vi "AcquireCameraImages.vi"() -> ()   [LabVIEW 2019]
uses:
  RecognitionResponse.ctl
  <vilib>/vision/Image Controls.llb/IMAQ Image.ctl
  <vilib>/vision/driver/IMAQdx.llb/IMAQdx Buffer Number Mode.ctl
  <vilib>/vision/driver/NI_Vision_Acquisition_Software.lvlib
panel:
  in  "Check face":bool
  out "error out":errorcluster
  out "Faces sent":i32
  out "value":T1={"probability"=0.0, "recognized_class"="127.0.0.1", "outcome"="false"}
  out "Image out":T2(plugin-control)
  out "Processing Frame Rate":dbl
  out "Acquired Frame Rate":dbl
  in  "Stop":bool
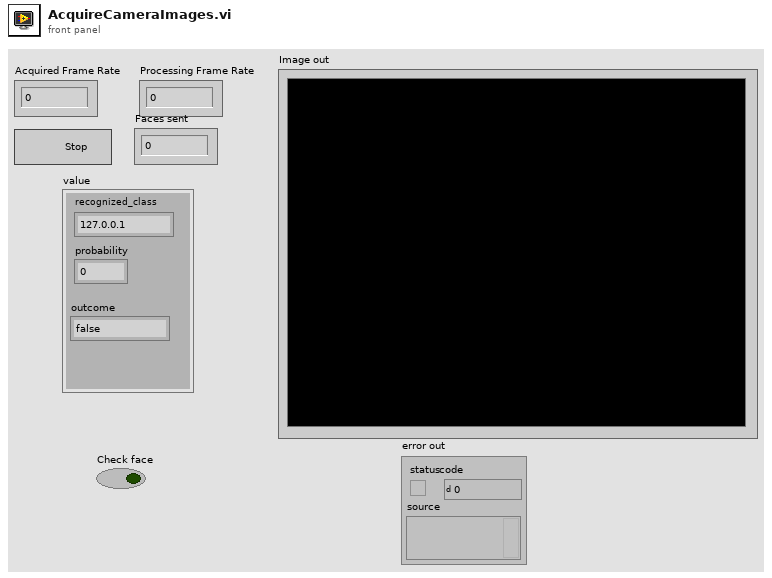
[diagram p1: front panel]
types:
  T1 = typedef "RecognitionResponse.ctl" = cluster{"probability":dbl, "recognized_class":string, "outcome":string}
  T2 = typedef "IMAQ Image.ctl" = refnum<image>
  T3 = typedef "IMAQ Object Tracking Session.ctl" = refnum<k20>
  T4 = typedef "IMAQdx.ctl" = refnum<k21>
  T5 = typedef "NI_Vision_Acquisition_Software.lvlib/IMAQdx Buffer Number Mode.ctl" = enum32{"Next", "Last", "Buffer Number", "Every", "Last New"}
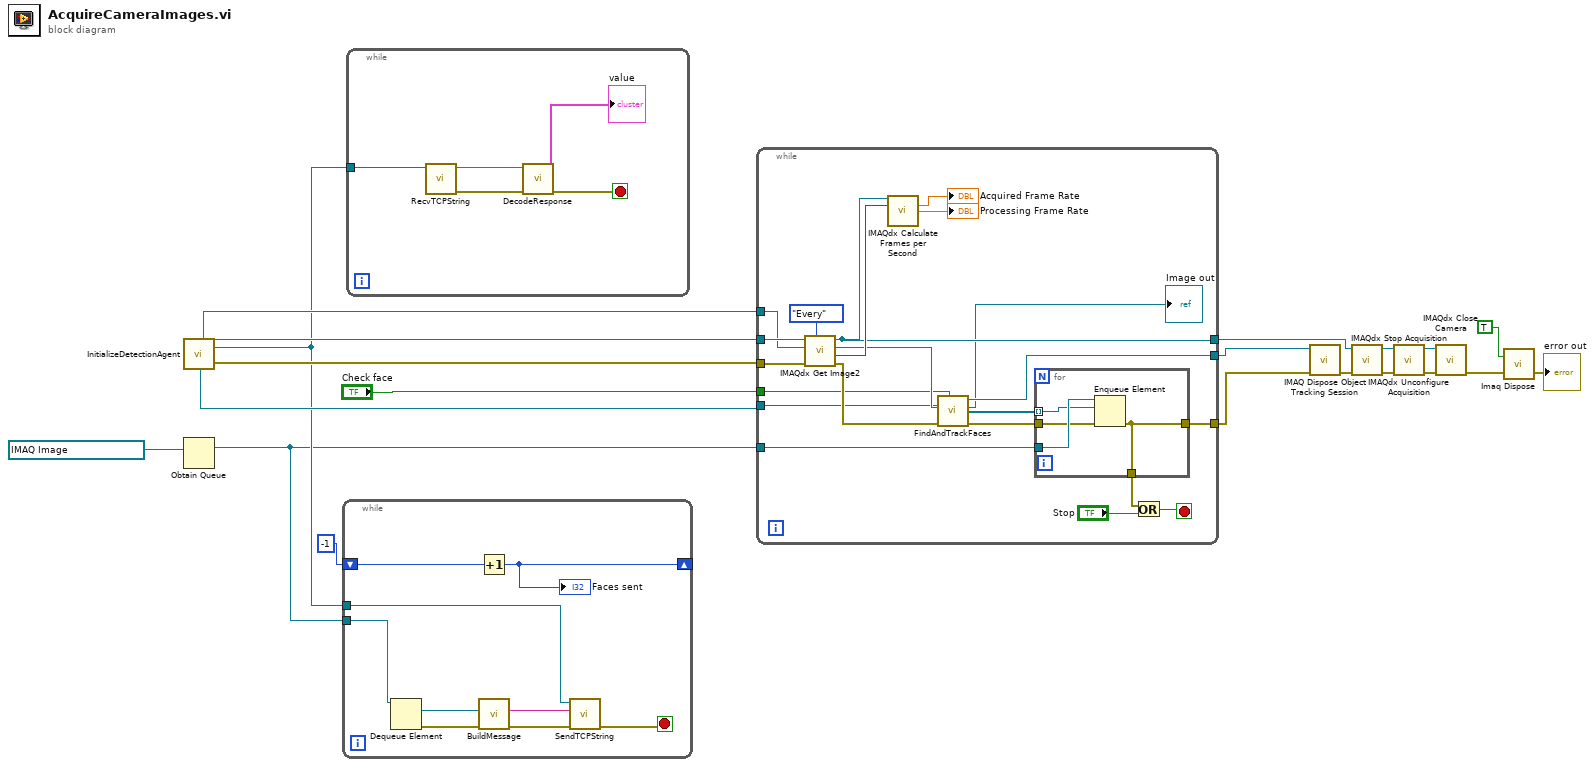
[diagram p0: block diagram]
diagram:
  n1 = call "InitializeDetectionAgent.vi"() -> ("error out"=w8:errorcluster, "Object Tracking Session Out"=w9:T3, "Session Out"=w10:T4, "connection ID"=w6:refnum<k5>, "Aquisition Image"=w11:T2)  [unwired: 6 in]
  n2 = Obtain Queue(element data type=T2 refnum ("Image type")) -> (queue out=w5:refnum<queue>)  [unwired: 4 in, 2 out]
  n3 = while {
    tunnel: w5 -> [w29]
    shift-right: [w21] -> _
    shift-left: -1 -> [w27]
    tunnel: w6 -> [w25]
    stop <- w22 stop-if-true
    n4 = Dequeue Element(queue=w29) -> (element=w28:T2, error out=w26:errorcluster)  [unwired: 2 in, 2 out]
    n5 = Increment(x=w27) -> (x+1=w21:i32)
    "Faces sent" <- w21
    n6 = call "BuildMessage.vi"("error in"=w26, "Image"=w28) -> ("error out"=w24:errorcluster, "JSON string"=w23:string)  [unwired: 7 in, 1 out]
    n7 = call "SendTCPString.vi"("error in (no error)"=w24, "String"=w23, "TCP Network Connection in"=w25) -> ("error out"=w22:errorcluster)  [unwired: 8 in]
  }
  n8 = while {
    tunnel: w6 -> [w32]
    stop <- w30 stop-if-true
    n9 = call "RecvTCPString.vi"("TCP Network Connection in"=w32) -> ("error out"=w31:errorcluster, "data out"=w34:string)  [unwired: 9 in]
    n10 = call "DecodeResponse.vi"("error in (no error)"=w31, "data in"=w34) -> ("error out"=w30:errorcluster, "RecognitionResponse"=→"value":T1)  [unwired: 8 in]
  }
  n11 = while {
    tunnel: [w50] -> w15
    tunnel: w8 -> [w55]
    tunnel: w10 -> [w54]
    tunnel: w11 -> [w52]
    tunnel: [w45] -> w13
    tunnel: w9 -> [w42]
    tunnel: w5 -> [w41]
    tunnel: [w39] -> w3
    tunnel: "Check face" -> [w35]
    stop <- w36 stop-if-true
    n12 = call <vilib>:"IMAQdx Get Image2.vi"("Buffer Number Mode (Next)"=IMAQdx_Buffer_Number_Mode."Every" ("Buffer Number Mode"), "error in"=w55, "Image In"=w52, "Session In"=w54) -> ("error out"=w46:errorcluster, "Buffer Number Out"=w51:u32, "Image Out"=w47:T2, "Session Out"=w50:T4)  [unwired: 4 in]
    n13 = call <vilib>:"IMAQdx Calculate Frames per Second.vi"("Session In"=w50, "Buffer Number"=w51) -> ("Acquired Frames per Second"=→"Acquired Frame Rate":dbl, "Processed Frames per Second"=→"Processing Frame Rate":dbl)  [unwired: 7 in, 5 out]
    n14 = call "FindAndTrackFaces.vi"("Check face"=w35, "error in (no error)"=w46, "Image in"=w47, "Object Tracking Session In"=w42) -> ("error out"=w43:errorcluster, "Face Images"=w44:T2[], "Image out"=→"Image out":T2, "Object Tracking Session Out"=w45:T3)  [unwired: 4 in]
    n15 = for {
      tunnel: w44 -> [w58] mode=indexing
      tunnel: w43 -> [w57]
      tunnel: w41 -> [w59]
      tunnel: [w56] -> w39
      tunnel: [w56] -> w37
      n16 = Enqueue Element(queue=w59, element=w58, error in (no error)=w57) -> (error out=w56:errorcluster)  [unwired: 1 in, 2 out]
    }
    n17 = Or(x=w37, y="Stop") -> (x .or. y?=w36:bool)
  }
  n18 = call "IMAQ Dispose Object Tracking Session"("error in (no error)"=w3, "Object Tracking Session"=w13) -> ("error out"=w12:errorcluster)  [unwired: 9 in]
  n19 = call <vilib>:"IMAQdx Stop Acquisition.vi"("error in"=w12, "Session In"=w15) -> ("error out"=w17:errorcluster, "Session Out"=w18:T4)  [unwired: 8 out]
  n20 = call <vilib>:"IMAQdx Unconfigure Acquisition.vi"("error in"=w17, "Session In"=w18) -> ("error out"=w20:errorcluster, "Session Out"=w19:T4)  [unwired: 8 out]
  n21 = call <vilib>:"IMAQdx Close Camera.vi"("error in"=w20, "Session In"=w19) -> ("error out"=w16:errorcluster)  [unwired: 9 out]
  n22 = call "Imaq Dispose"("All Images? (No)"=TRUE, "error in (no error)"=w16) -> ("error out"=→"error out":errorcluster)  [unwired: 4 in]
